vi "Item_OnCommand.vi"(10 "Command ID":string, 11 "Object":T1) -> ()   [LabVIEW 2020, in "Message Maker Provider.lvlib"]
uses:
  Message Maker Provider.lvlib
  _Message Maker/Message Maker.lvlib
  AFPP Shared/AFPP Shared.lvlib
  <vilib>/ErrorRing/Error Ring.xnode
  AFPP Shared/Validation Mode.ctl
  <vilib>/Utility/error.llb/Error Cluster From Error Code.vi
  <resource>/Framework/Providers/API/ItemRef.ctl
panel:
  out "error out":errorcluster
  in  "error in":errorcluster
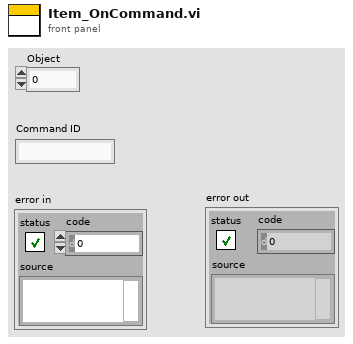
[diagram p1: front panel]
types:
  T1 = typedef "ItemRef.ctl" = u64
  T2 = typedef "AFPP Shared.lvlib/Validation Mode.ctl" = enum16{"An Actor Library", "A Target Tag"}
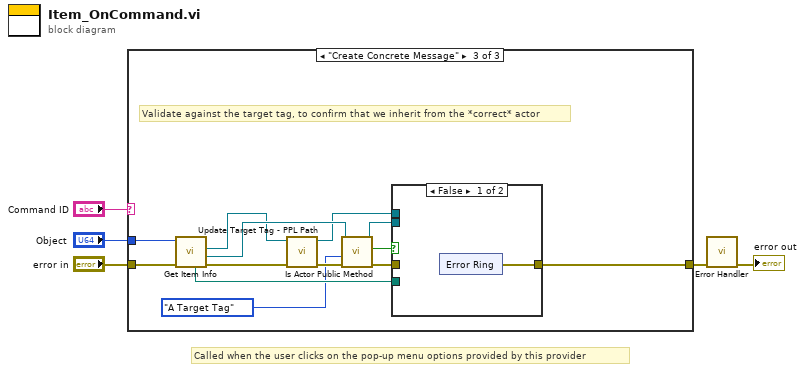
[diagram p0: block diagram]
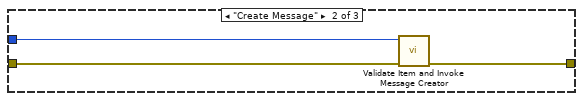
[diagram p3: hidden frame]
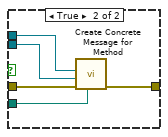
[diagram p4: hidden frame]
diagram:
  # "Called when the user clicks on the pop-up menu options provided by this provider"
  n1 = case shown="\"Create Concrete Message\"" "Command ID" {
    tunnel: "error in" -> [w6 w9 w19]
    tunnel: [w6 w8 w22] -> w2
    tunnel: "Object" -> [_ w7 w21]
    frame Default {
    }
    frame "Create Message" {
      n2 = call "Validate Item and Invoke Message Creator.vi"("error in (no error)"=w9, "Object"=w7) -> ("error out"=w8:errorcluster)  [unwired: 9 in]
    }
    frame "Create Concrete Message" {
      # "Validate against the target tag, to confirm that we inherit from the *correct* actor"
      n3 = call "Get Item Info.vi"("error in (no error)"=w19, "Object"=w21) -> ("error out"=w17:errorcluster, "Item Refnum"=w14:refnum<vi>, "Target"=w12:refnum<vi>, "Project Path"=w20:path)  [unwired: 5 in, 1 out]
      n4 = call "Update Target Tag - PPL Path.vi"("error in (no error)"=w17, "Target"=w12) -> ("error out"=w18:errorcluster, "dup Target"=w11:refnum<vi>)  [unwired: 7 in, 1 out]
      n5 = call "Is Actor Public Method.vi"("error in (no error)"=w18, "Validation"=Validation_Mode."A Target Tag", "ProjectItem in"=w14) -> ("error out"=w16:errorcluster, "Is Actor Public Method"=w15:bool, "ProjectItem out"=w13:refnum<vi>)  [unwired: 5 in, 1 out]
      n6 = case shown="False" w15 {
        tunnel: [w23 w33] -> w22
        tunnel: w20 -> [_ w32]
        tunnel: w11 -> [_ w31]
        tunnel: w13 -> [_ w30]
        tunnel: w16 -> [_ w29]
        frame False {
          n7 = xnode "Error Ring"() -> ("error out"=w23:errorcluster)
        }
        frame True {
          n8 = call "Create Concrete Message for Method.vi"("Project Path"=w32, "error in (no error)"=w29, "Item Refnum"=w30, "Target"=w31) -> ("error out"=w33:errorcluster)  [unwired: 7 in]
        }
      }
    }
  }
  n9 = call "Error Handler.vi"("error in (no error)"=w2) -> ("error out"=→"error out":errorcluster)  [unwired: 10 in]
